vi "绘制预览图片.vi"(8 "error in (no error)":errorcluster caption="错误输入（无错误）", 11 "程序 输入":refnum<class "程序.lvclass">) -> (0 "error out":errorcluster caption="错误输出", 3 "程序 输出":refnum<class "程序.lvclass">)   [LabVIEW 2020, in "程序.lvclass"]
uses:
  <vilib>/Utility/miscctls.llb/LVPoint32TypeDef.ctl
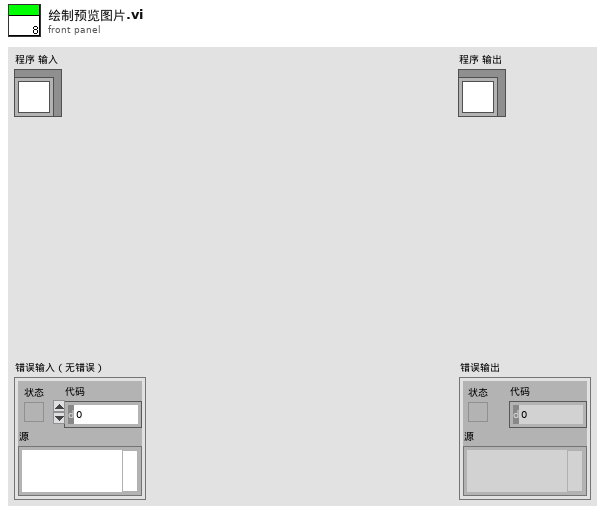
[diagram p1: front panel]
types:
  T1 = typedef "LVPoint32TypeDef.ctl" = cluster{"Horizontal":i32, "Vertical":i32}
  T2 = typedef "LVPositionTypeDef.ctl" = cluster{"Left":i32, "Top":i32}
  T3 = typedef "imagedata.ctl" = cluster{"image type":i32, "image depth":i32, "image":u8[], "mask":u8[], "colors":u32[], "Rectangle":cluster{"left":i16, "top":i16, "right":i16, "bottom":i16}}
  T4 = cluster{"图片":picture, "名称":string, "文本程序":string, "关键字":string, "image data":T3}[][]
  T5 = typedef "LVBoundsTypeDef.ctl" = cluster{"Width":u32, "Height":u32}
  T6 = cluster{"图片":picture, "名称":string, "文本程序":string, "关键字":string, "image data":T3}
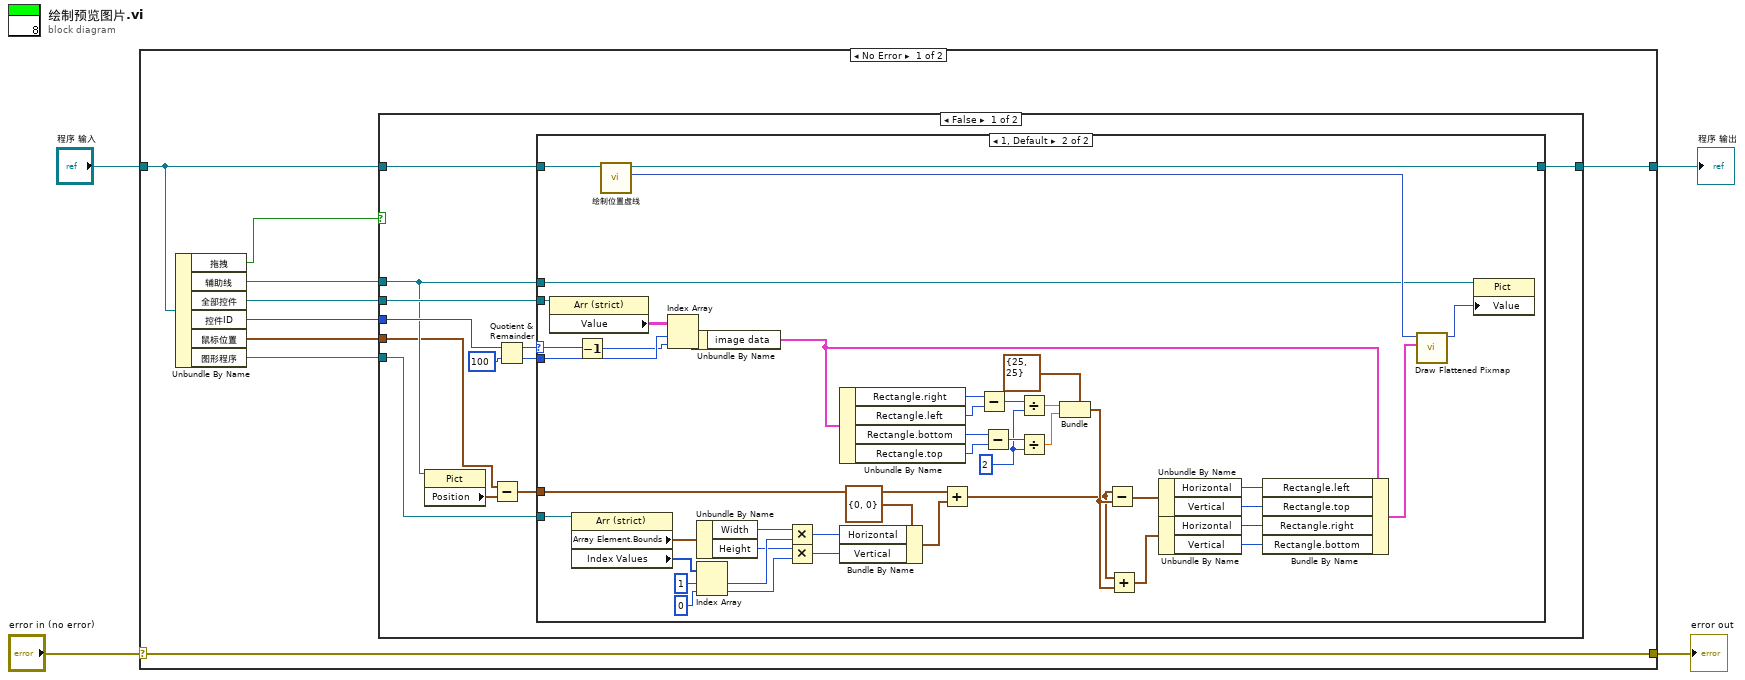
[diagram p0: block diagram]
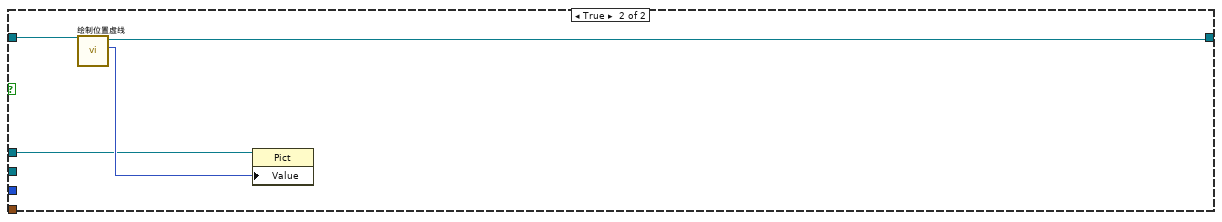
[diagram p3: hidden frame]
diagram:
  n1 = case shown="No Error" "error in (no error)" {
    selector: "error in (no error)" -> [w13 w77]
    tunnel: [w13 w77] -> w1
    tunnel: [w9 w76] -> w4
    tunnel: "程序 输入" -> [w10 w76]
    frame No Error {
      n2 = Unbundle By Name(w10) -> ("拖拽"=w5:bool, "辅助线"=w8:refnum<vi>, "全部控件"=w11:refnum<vi>, "控件ID"=w12:u32, "鼠标位置"=w7:T1, "图形程序"=w6:refnum<vi>)
      n3 = case shown="False" w5 {
        tunnel: w12 -> [w25 _]
        tunnel: w11 -> [w23 _]
        tunnel: w10 -> [w21 w75]
        tunnel: [w20 w74] -> w9
        tunnel: w8 -> [w19 w72]
        tunnel: w7 -> [w18 _]
        tunnel: w6 -> [w14 _]
        frame False {
          n4 = property class="Pict"(reference=w19) -> ("Position"=w17:T2)  [unwired: 1 in, 2 out]
          n5 = Subtract(x=w18, y=w17) -> (x-y=w16:T1)
          n6 = Quotient & Remainder(x=w25, y=u32 100) -> (x-y*floor(x/y)=w22:u32, floor(x/y)=w15:u32)
          n7 = case shown="1, Default" w22 {
            selector: w22 -> [_ w68]
            tunnel: w19 -> [_ w56]
            tunnel: w23 -> [_ w69]
            tunnel: w16 -> [_ w29]
            tunnel: w21 -> [w26 w59]
            tunnel: [w26 w58] -> w20
            tunnel: w15 -> [_ w55]
            tunnel: w14 -> [_ w42]
            frame 0 {
            }
            frame 1, Default {
              w47 = i16 2 ("y")
              n8 = property class="Arr (strict)"(reference=w69) -> ("Value"=w71:T4)  [unwired: 1 in, 2 out]
              n9 = property class="Arr (strict)"(reference=w42) -> ("Array Element.Bounds"=w41:T5, "Index Values"=w40:u32[])  [unwired: 1 in, 2 out]
              n10 = Decrement(x=w68) -> (x-1=w54:u32)
              n11 = call-dynamic "绘制位置虚线.vi"("程序 输入"=w59) -> ("new picture"=w57:picture, "程序 输出"=w58:refnum<class "程序.lvclass">)  [unwired: 8 in, 1 out]
              n12 = Index Array(array=w71, index (row)=w55, index (col)=w54) -> (element=w70:T6)
              n13 = Unbundle By Name(w70) -> ("image data"=w27:T3)
              n14 = Unbundle By Name(w41) -> ("Width"=w37:u32, "Height"=w35:u32)
              n15 = Index Array(array=w40, index #1=1 ("索引"), index #2=0 ("索引")) -> (element #1=w36:u32, element #2=w34:u32)
              n16 = Multiply(x=w37, y=w36) -> (x*y=w32:u32)
              n17 = Multiply(x=w35, y=w34) -> (x*y=w31:u32)
              n18 = Unbundle By Name(w27) -> ("Rectangle.right"=w53:i16, "Rectangle.left"=w52:i16, "Rectangle.bottom"=w51:i16, "Rectangle.top"=w50:i16)
              n19 = Bundle By Name(cluster=T1 {"Horizontal"=0, "Vertical"=0} ("鼠标位置"), "Horizontal"=w32, "Vertical"=w31) -> (w30:T1)
              n20 = Add(x=w29, y=w30) -> (x+y=w28:T1)
              n21 = Subtract(x=w53, y=w52) -> (x-y=w49:i16)
              n22 = Subtract(x=w51, y=w50) -> (x-y=w48:i16)
              n23 = Divide(x=w49, y=w47) -> (x/y=w46:dbl)
              n24 = Divide(x=w48, y=w47) -> (x/y=w45:dbl)
              n25 = Bundle(cluster=T1 {"Horizontal"=25, "Vertical"=25} ("y"), "Horizontal"=w46, "Vertical"=w45) -> (w43:T1)
              n26 = Subtract(x=w28, y=w43) -> (x-y=w67:T1)
              n27 = Add(x=w28, y=w43) -> (x+y=w66:T1)
              n28 = Unbundle By Name(w67) -> ("Horizontal"=w64:i32, "Vertical"=w63:i32)
              n29 = Unbundle By Name(w66) -> ("Horizontal"=w62:i32, "Vertical"=w61:i32)
              n30 = Bundle By Name(cluster=w27, "Rectangle.left"=w64, "Rectangle.top"=w63, "Rectangle.right"=w62, "Rectangle.bottom"=w61) -> (w65:T3)
              n31 = call <vilib>:"Draw Flattened Pixmap.vi"("image data"=w65, "picture"=w57) -> ("new picture"=w60:picture)  [unwired: 7 in]
              n32 = property class="Pict"(reference=w56, "Value"=w60) -> ()  [unwired: 1 in, 2 out]
            }
          }
        }
        frame True {
          n33 = call-dynamic "绘制位置虚线.vi"("程序 输入"=w75) -> ("new picture"=w73:picture, "程序 输出"=w74:refnum<class "程序.lvclass">)  [unwired: 8 in, 1 out]
          n34 = property class="Pict"(reference=w72, "Value"=w73) -> ()  [unwired: 1 in, 2 out]
        }
      }
    }
    frame Error {
    }
  }
  "error out" <- w1
  "程序 输出" <- w4
